vi "FGV.vi"(9 "Enum":T1, 10 "Data in":sgl format="%#_13g") -> (2 "Output Array":sgl[](array[numeric]))   [LabVIEW 2015]
uses:
  DBEnum.ctl
  main_data_typedef.ctl
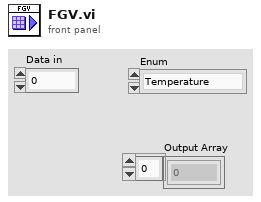
[diagram p1: front panel]
types:
  T1 = typedef "DBEnum.ctl" = enum16{"Temperature", "HeartRate", "XAccelero", "YAccelero", "ZAccelero"}
  T2 = typedef "main_data_typedef.ctl" = cluster{"HeartRate":sgl[], "Temperature":sgl[], "XAccelero":sgl[], "YAccelero":sgl[], "ZAccelero":sgl[]}
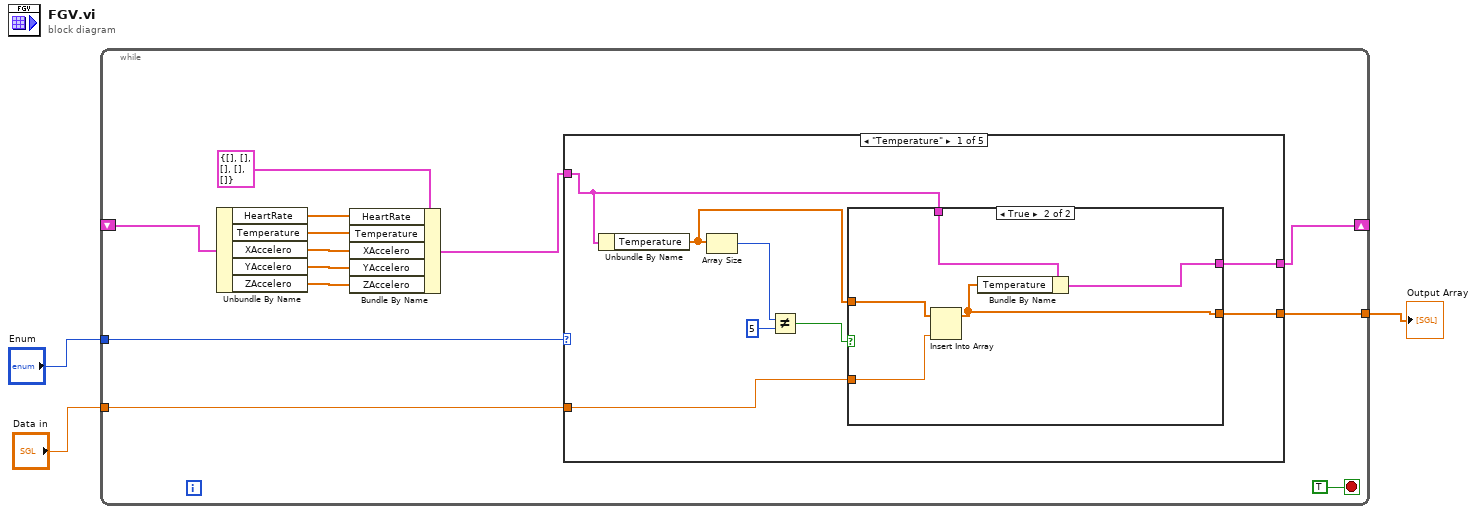
[diagram p0: block diagram]
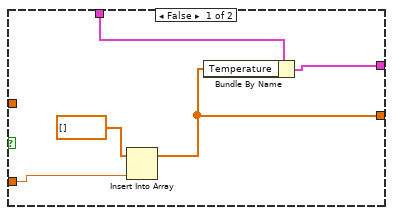
[diagram p2: hidden frame]
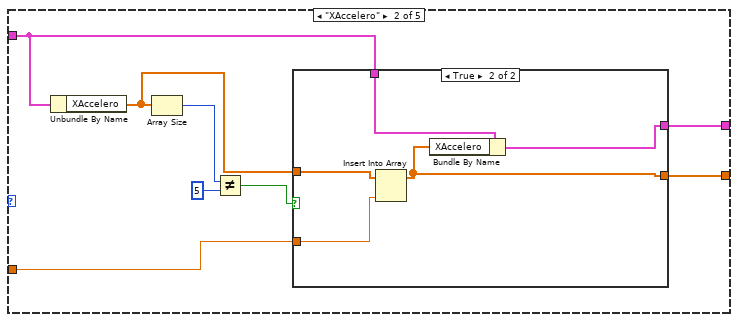
[diagram p3: hidden frame]
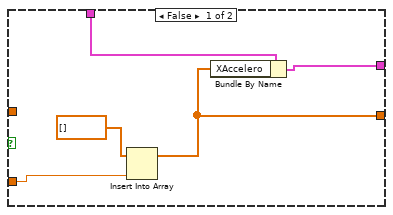
[diagram p4: hidden frame]
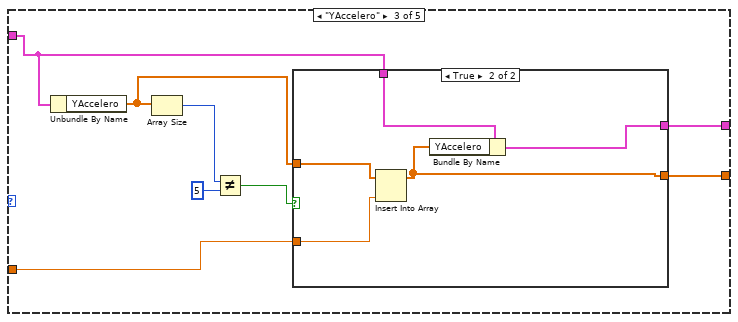
[diagram p5: hidden frame]
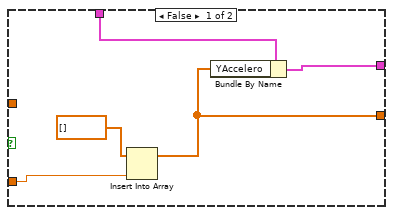
[diagram p6: hidden frame]
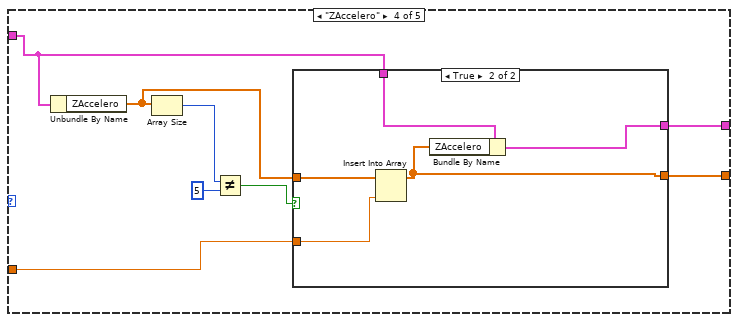
[diagram p7: hidden frame]
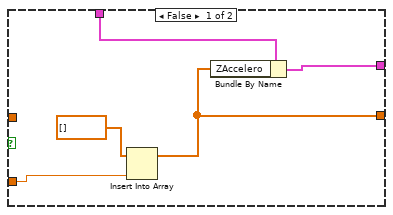
[diagram p8: hidden frame]
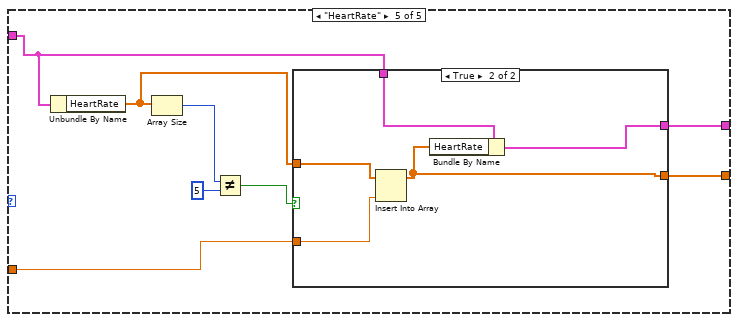
[diagram p9: hidden frame]
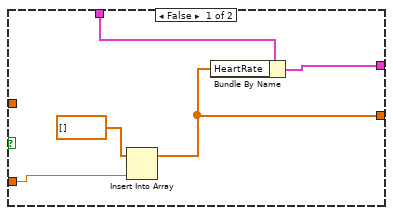
[diagram p10: hidden frame]
diagram:
  n1 = while {
    tunnel: "Data in" -> [w15]
    tunnel: "Enum" -> [w14]
    tunnel: [w12] -> w1
    shift-right: [w13] -> _
    shift-left: _ -> [w10]
    stop <- TRUE stop-if-true
    n2 = Unbundle By Name(w10) -> ("HeartRate"=w8:sgl[], "Temperature"=w7:sgl[], "XAccelero"=w6:sgl[], "YAccelero"=w5:sgl[], "ZAccelero"=w4:sgl[])
    n3 = Bundle By Name(cluster=T2 {"HeartRate"=[], "Temperature"=[], "XAccelero"=[], "YAccelero"=[], "ZAccelero"=[]} ("Data"), "HeartRate"=w8, "Temperature"=w7, "XAccelero"=w6, "YAccelero"=w5, "ZAccelero"=w4) -> (w11:T2)
    n4 = case shown="\"Temperature\"" w14 {
      tunnel: w15 -> [w20 w39 w56 w74 w92]
      tunnel: [w21 w37 w57 w75 w93] -> w13
      tunnel: [w19 w38 w55 w73 w91] -> w12
      tunnel: w11 -> [w18 w36 w54 w72 w90]
      frame "Temperature" {
        n5 = Unbundle By Name(w18) -> ("Temperature"=w17:sgl[])
        n6 = Array Size(array=w17) -> (size(s)=w24:i32)
        n7 = Not Equal?(x=w24, y=5) -> (x != y?=w22:bool)
        n8 = case shown="True" w22 {
          tunnel: w18 -> [w29 w34]
          tunnel: [w26 w33] -> w21
          tunnel: w20 -> [w27 w32]
          tunnel: [w25 w31] -> w19
          tunnel: w17 -> [_ w30]
          frame False {
            n9 = Insert Into Array(array=sgl[] [], new element=w27) -> (w25:sgl[])  [unwired: 1 in]
            n10 = Bundle By Name(cluster=w29, "Temperature"=w25) -> (w26:T2)
          }
          frame True {
            n11 = Insert Into Array(array=w30, new element=w32) -> (w31:sgl[])  [unwired: 1 in]
            n12 = Bundle By Name(cluster=w34, "Temperature"=w31) -> (w33:T2)
          }
        }
      }
      frame "XAccelero" {
        n13 = Unbundle By Name(w36) -> ("XAccelero"=w35:sgl[])
        n14 = Array Size(array=w35) -> (size(s)=w42:i32)
        n15 = Not Equal?(x=w42, y=5) -> (x != y?=w40:bool)
        n16 = case shown="True" w40 {
          tunnel: [w43 w49] -> w37
          tunnel: w39 -> [w46 w52]
          tunnel: [w45 w51] -> w38
          tunnel: w36 -> [w44 w50]
          tunnel: w35 -> [_ w48]
          frame False {
            n17 = Insert Into Array(array=sgl[] [], new element=w46) -> (w45:sgl[])  [unwired: 1 in]
            n18 = Bundle By Name(cluster=w44, "XAccelero"=w45) -> (w43:T2)
          }
          frame True {
            n19 = Insert Into Array(array=w48, new element=w52) -> (w51:sgl[])  [unwired: 1 in]
            n20 = Bundle By Name(cluster=w50, "XAccelero"=w51) -> (w49:T2)
          }
        }
      }
      frame "YAccelero" {
        n21 = Unbundle By Name(w54) -> ("YAccelero"=w53:sgl[])
        n22 = Array Size(array=w53) -> (size(s)=w60:i32)
        n23 = Not Equal?(x=w60, y=5) -> (x != y?=w58:bool)
        n24 = case shown="True" w58 {
          tunnel: w54 -> [w65 w70]
          tunnel: [w62 w69] -> w57
          tunnel: w56 -> [w63 w68]
          tunnel: [w61 w67] -> w55
          tunnel: w53 -> [_ w66]
          frame False {
            n25 = Insert Into Array(array=sgl[] [], new element=w63) -> (w61:sgl[])  [unwired: 1 in]
            n26 = Bundle By Name(cluster=w65, "YAccelero"=w61) -> (w62:T2)
          }
          frame True {
            n27 = Insert Into Array(array=w66, new element=w68) -> (w67:sgl[])  [unwired: 1 in]
            n28 = Bundle By Name(cluster=w70, "YAccelero"=w67) -> (w69:T2)
          }
        }
      }
      frame "ZAccelero" {
        n29 = Unbundle By Name(w72) -> ("ZAccelero"=w71:sgl[])
        n30 = Array Size(array=w71) -> (size(s)=w78:i32)
        n31 = Not Equal?(x=w78, y=5) -> (x != y?=w76:bool)
        n32 = case shown="True" w76 {
          tunnel: w72 -> [w83 w88]
          tunnel: [w80 w87] -> w75
          tunnel: w74 -> [w81 w86]
          tunnel: [w79 w85] -> w73
          tunnel: w71 -> [_ w84]
          frame False {
            n33 = Insert Into Array(array=sgl[] [], new element=w81) -> (w79:sgl[])  [unwired: 1 in]
            n34 = Bundle By Name(cluster=w83, "ZAccelero"=w79) -> (w80:T2)
          }
          frame True {
            n35 = Insert Into Array(array=w84, new element=w86) -> (w85:sgl[])  [unwired: 1 in]
            n36 = Bundle By Name(cluster=w88, "ZAccelero"=w85) -> (w87:T2)
          }
        }
      }
      frame "HeartRate" {
        n37 = Unbundle By Name(w90) -> ("HeartRate"=w89:sgl[])
        n38 = Array Size(array=w89) -> (size(s)=w96:i32)
        n39 = Not Equal?(x=w96, y=5) -> (x != y?=w94:bool)
        n40 = case shown="True" w94 {
          tunnel: w90 -> [w101 w106]
          tunnel: [w98 w105] -> w93
          tunnel: w92 -> [w99 w104]
          tunnel: [w97 w103] -> w91
          tunnel: w89 -> [_ w102]
          frame False {
            n41 = Insert Into Array(array=sgl[] [], new element=w99) -> (w97:sgl[])  [unwired: 1 in]
            n42 = Bundle By Name(cluster=w101, "HeartRate"=w97) -> (w98:T2)
          }
          frame True {
            n43 = Insert Into Array(array=w102, new element=w104) -> (w103:sgl[])  [unwired: 1 in]
            n44 = Bundle By Name(cluster=w106, "HeartRate"=w103) -> (w105:T2)
          }
        }
      }
    }
  }
  "Output Array" <- w1
